vi "SMO.Example.A.vi"(8 "error in (no error)":errorcluster, 11 "SMO.Example":refnum<class "SMO.TopLevel.lvclass">) -> (0 "error out":errorcluster, 2 "Nested Dependency Name":string, 3 "SMO.Example out":refnum<class "SMO.TopLevel.lvclass">)   [LabVIEW 2021, in "SMO.TopLevel.lvclass"]
doc: "---------------------------------------------------------------\nJKI State Machine Objects™\nhttp://jki.net/state-machine-objects/\nCopyright (C) 2005-2015, JKI <info@jki.net>\nALL RIGHTS RESERVED"
uses:
  SMO.TopLevel.lvclass
  SMO.TopLevel.lvclass/SMO.TopLevel.ctl
  src/SMO/SMO.lvclass
  SMO.A/SMO.A.lvclass
  C:/Repositories/SMO/src/SMO/SMO.lvclass
  C:/Repositories/SMO/tests/_test-support-SMOs/SMO.A/SMO.A.lvclass
panel:
  # "For instructions on how to use the JKI State Machine Objects, examples and video tutorials, visit:\nhttp://jki.net/state-machine-objects/\n\nJKI State Machine Objects™\nhttp://jki.net/state-machine-objects/\nCopyright (C) 2005-2015, JKI <info@jki.net>\nALL RIGHTS RESERVED"
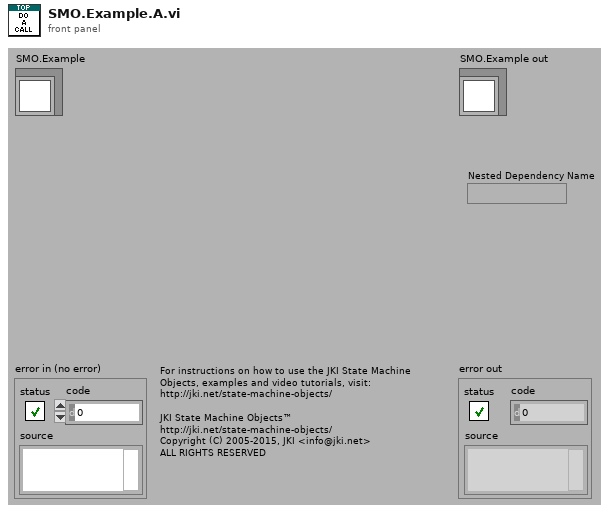
[diagram p1: front panel]
types:
  T1 = typedef "SMO.TopLevel.lvclass/Dependencies--Cluster.ctl" = cluster{"A":refnum<class "SMO.A.lvclass">, "A2":refnum<class "SMO.A.lvclass">, "A3":refnum<class "SMO.A.lvclass">, "A4":refnum<class "SMO.A.lvclass">}
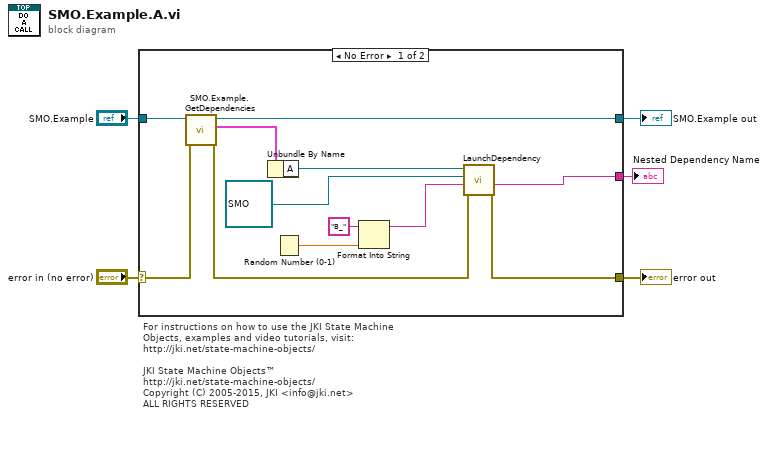
[diagram p0: block diagram]
diagram:
  # "For instructions on how to use the JKI State Machine Objects, examples and video tutorials, visit:\nhttp://jki.net/state-machine-objects/\n\nJKI State Machine Objects™\nhttp://jki.net/state-machine-objects/\nCopyright (C) 2005-2015, JKI <info@jki.net>\nALL RIGHTS RESERVED"
  n1 = case shown="No Error" "error in (no error)" {
    selector: "error in (no error)" -> [w16 w18]
    tunnel: "SMO.Example" -> [w17 w19]
    tunnel: [w12 w18] -> w4
    tunnel: [w14 w19] -> w3
    tunnel: [w11 _] -> w1
    frame No Error {
      n2 = call "SMO.Example.GetDependencies.vi"("error in (no error)"=w16, "SMO.Example"=w17) -> ("error out"=w13:errorcluster, "Dependencies"=w15:T1, "SMO.Example out"=w14:refnum<class "SMO.TopLevel.lvclass">)  [unwired: 7 in]
      n3 = Unbundle By Name(w15) -> ("A"=w8:refnum<class "SMO.A.lvclass">)
      n4 = Random Number (0-1)() -> (number: 0 to 1=w9:dbl)
      n5 = Format Into String(initial string="B_", w9) -> (resulting string=w10:string)  [unwired: 2 in, 1 out]
      n6 = call "LaunchDependency.vi"("error in (no error)"=w13, "Dependency Name"=w10, "Dependency Type"=refnum<class "SMO.lvclass"> refnum ("smo.lvlib:SMO.lvclass"), "SMO in"=w8) -> ("error out"=w12:errorcluster, "Unique Name"=w11:string)  [unwired: 4 in, 2 out]
    }
    frame Error {
    }
  }
  "error out" <- w4
  "SMO.Example out" <- w3
  "Nested Dependency Name" <- w1
